vi "Periodic Tasks.vi"(8 "error in":errorcluster) -> ()   [LabVIEW 2014]
doc: "This VI runs in parallel to other tasks. It can contain as many user-defined periodic loops as you need. These can carry out PID or other sorts of timed response."
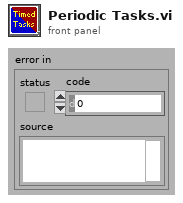
[diagram p1: front panel]
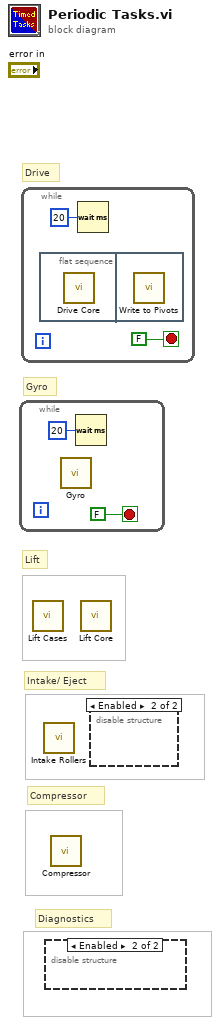
[diagram p0: block diagram]
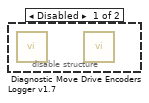
[diagram p2: hidden frame]
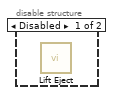
[diagram p3: hidden frame]
diagram:
  # "Drive"
  # "Gyro"
  # "Diagnostics"
  # "Compressor"
  # "Intake/ Eject"
  # "Lift"
  n1 = while {
    stop <- FALSE stop-if-true
    n2 = call "Gyro.vi"() -> ()  [unwired: 12 in]
    n3 = Wait (ms)(milliseconds to wait=u32 20) -> ()  [unwired: 1 out]
  }
  n4 = while {
    stop <- FALSE stop-if-true
    n5 = flat-sequence {
      frame #0 {
        n6 = call "Drive Core.vi"() -> ()  [unwired: 12 in]
      }
      frame #1 {
        n7 = call "Write to Pivots.vi"() -> ()  [unwired: 12 in]
      }
    }
    n8 = Wait (ms)(milliseconds to wait=u32 20) -> ()  [unwired: 1 out]
  }
  n9 = call "Lift Cases.vi"() -> ()  [unwired: 12 in]
  n10 = call "Intake Rollers.vi"() -> ()  [unwired: 12 in]
  n11 = disable-structure shown="Enabled" {
    frame Disabled {
      n12 = call "Diagnostic Logger v1.7.vi"() -> ()  [unwired: 1 in]
      n13 = call "Move Drive Encoders.vi"() -> ()  [unwired: 12 in]
    }
    frame Enabled {
    }
  }
  n14 = call "Compressor.vi"() -> ()  [unwired: 12 in]
  n15 = call "Lift Core.vi"() -> ()  [unwired: 12 in]
  n16 = disable-structure shown="Enabled" {
    frame Disabled {
      n17 = call "Lift Eject.vi"() -> ()  [unwired: 12 in]
    }
    frame Enabled {
    }
  }
